vi "DI&AO.vi"() -> ()   [LabVIEW 2016]
uses:
  <vilib>/rvi/Emulation/niFpgaGetClockAttributes.vi
  <vilib>/rvi/Emulation/niFpgaSctlEmulationGetInTimedLoop.vi
  <vilib>/rvi/Emulation/niFpgaEmulationReportErrorSimple.vi
  <vilib>/rvi/eio/common/nirviEmuTemplateMethod_errors.vi
  <vilib>/rvi/Emulation/niFpgaCriticalErrorInLSC.vi
  <vilib>/eio/EIONode/EIONode.xnode
panel:
  out "Boolean array":bool[](array[boolean])
  out "Mod2/DIO31:0":u32
  in  "Mod4/AO7":fxp<+/-,20,5>
  in  "Mod4/AO6":fxp<+/-,20,5>
  in  "Mod4/AO5":fxp<+/-,20,5>
  in  "Mod4/AO4":fxp<+/-,20,5>
  in  "Mod4/AO3":fxp<+/-,20,5>
  in  "Mod4/AO2":fxp<+/-,20,5>
  in  "Mod4/AO1":fxp<+/-,20,5>
  in  "Mod4/AO0":fxp<+/-,20,5>
  in  "Mod4/AO15":fxp<+/-,20,5>
  in  "Mod4/AO14":fxp<+/-,20,5>
  in  "Mod4/AO13":fxp<+/-,20,5>
  in  "Mod4/AO12":fxp<+/-,20,5>
  in  "Mod4/AO11":fxp<+/-,20,5>
  in  "Mod4/AO10":fxp<+/-,20,5>
  in  "Mod4/AO9":fxp<+/-,20,5>
  in  "Mod4/AO8":fxp<+/-,20,5>
  out "Mod2/DIO31":bool
  out "Mod2/DIO30":bool
  out "Mod2/DIO29":bool
  out "Mod2/DIO28":bool
  out "Mod2/DIO27":bool
  out "Mod2/DIO26":bool
  out "Mod2/DIO25":bool
  out "Mod2/DIO24":bool
  out "Mod2/DIO23":bool
  out "Mod2/DIO22":bool
  out "Mod2/DIO21":bool
  out "Mod2/DIO20":bool
  out "Mod2/DIO19":bool
  out "Mod2/DIO18":bool
  out "Mod2/DIO17":bool
  out "Mod2/DIO16":bool
  out "Mod2/DIO15":bool
  out "Mod2/DIO14":bool
  out "Mod2/DIO13":bool
  out "Mod2/DIO12":bool
  out "Mod2/DIO11":bool
  out "Mod2/DIO10":bool
  out "Mod2/DIO9":bool
  out "Mod2/DIO8":bool
  out "Mod2/DIO7":bool
  out "Mod2/DIO6":bool
  out "Mod2/DIO5":bool
  out "Mod2/DIO4":bool
  out "Mod2/DIO3":bool
  out "Mod2/DIO2":bool
  out "Mod2/DIO1":bool
  out "Mod2/DIO0":bool
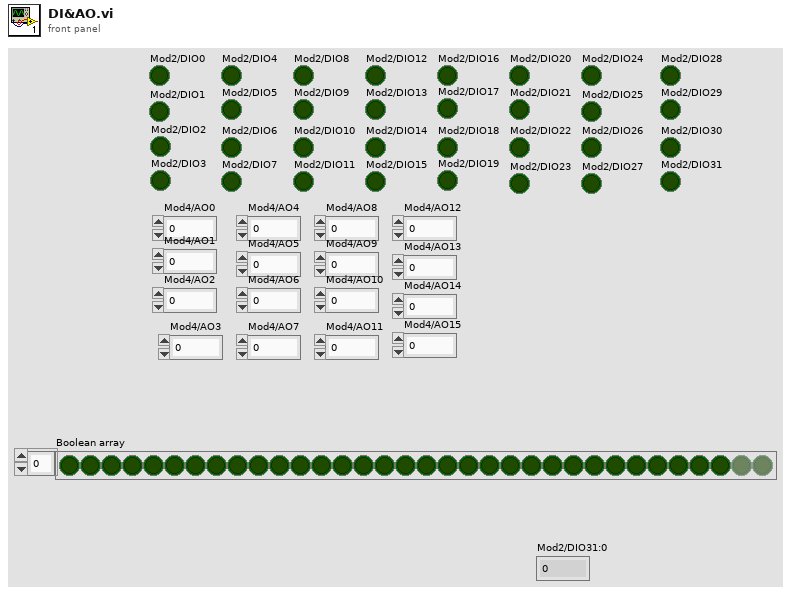
[diagram p1: front panel]
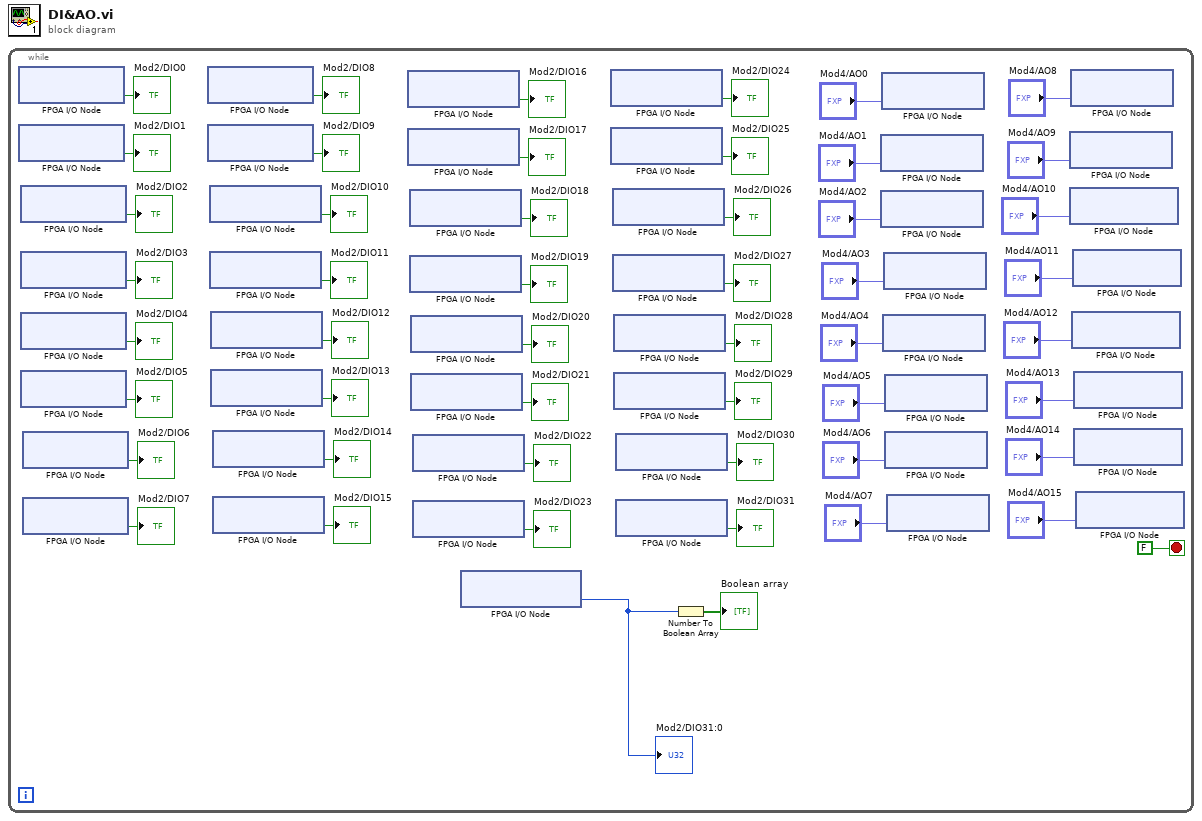
[diagram p0: block diagram]
diagram:
  n1 = while {
    stop <- FALSE stop-if-true
    n2 = xnode "FPGA I/O Node"() -> ("Mod2/DIO0"=→"Mod2/DIO0":bool)  [unwired: 1 in, 1 out]
    n3 = xnode "FPGA I/O Node"() -> ("Mod2/DIO1"=→"Mod2/DIO1":bool)  [unwired: 1 in, 1 out]
    n4 = xnode "FPGA I/O Node"() -> ("Mod2/DIO2"=→"Mod2/DIO2":bool)  [unwired: 1 in, 1 out]
    n5 = xnode "FPGA I/O Node"() -> ("Mod2/DIO3"=→"Mod2/DIO3":bool)  [unwired: 1 in, 1 out]
    n6 = xnode "FPGA I/O Node"() -> ("Mod2/DIO4"=→"Mod2/DIO4":bool)  [unwired: 1 in, 1 out]
    n7 = xnode "FPGA I/O Node"() -> ("Mod2/DIO5"=→"Mod2/DIO5":bool)  [unwired: 1 in, 1 out]
    n8 = xnode "FPGA I/O Node"() -> ("Mod2/DIO6"=→"Mod2/DIO6":bool)  [unwired: 1 in, 1 out]
    n9 = xnode "FPGA I/O Node"() -> ("Mod2/DIO7"=→"Mod2/DIO7":bool)  [unwired: 1 in, 1 out]
    n10 = xnode "FPGA I/O Node"() -> ("Mod2/DIO8"=→"Mod2/DIO8":bool)  [unwired: 1 in, 1 out]
    n11 = xnode "FPGA I/O Node"() -> ("Mod2/DIO9"=→"Mod2/DIO9":bool)  [unwired: 1 in, 1 out]
    n12 = xnode "FPGA I/O Node"() -> ("Mod2/DIO10"=→"Mod2/DIO10":bool)  [unwired: 1 in, 1 out]
    n13 = xnode "FPGA I/O Node"() -> ("Mod2/DIO11"=→"Mod2/DIO11":bool)  [unwired: 1 in, 1 out]
    n14 = xnode "FPGA I/O Node"() -> ("Mod2/DIO12"=→"Mod2/DIO12":bool)  [unwired: 1 in, 1 out]
    n15 = xnode "FPGA I/O Node"() -> ("Mod2/DIO13"=→"Mod2/DIO13":bool)  [unwired: 1 in, 1 out]
    n16 = xnode "FPGA I/O Node"() -> ("Mod2/DIO14"=→"Mod2/DIO14":bool)  [unwired: 1 in, 1 out]
    n17 = xnode "FPGA I/O Node"() -> ("Mod2/DIO15"=→"Mod2/DIO15":bool)  [unwired: 1 in, 1 out]
    n18 = xnode "FPGA I/O Node"() -> ("Mod2/DIO16"=→"Mod2/DIO16":bool)  [unwired: 1 in, 1 out]
    n19 = xnode "FPGA I/O Node"() -> ("Mod2/DIO17"=→"Mod2/DIO17":bool)  [unwired: 1 in, 1 out]
    n20 = xnode "FPGA I/O Node"() -> ("Mod2/DIO18"=→"Mod2/DIO18":bool)  [unwired: 1 in, 1 out]
    n21 = xnode "FPGA I/O Node"() -> ("Mod2/DIO19"=→"Mod2/DIO19":bool)  [unwired: 1 in, 1 out]
    n22 = xnode "FPGA I/O Node"() -> ("Mod2/DIO20"=→"Mod2/DIO20":bool)  [unwired: 1 in, 1 out]
    n23 = xnode "FPGA I/O Node"() -> ("Mod2/DIO21"=→"Mod2/DIO21":bool)  [unwired: 1 in, 1 out]
    n24 = xnode "FPGA I/O Node"() -> ("Mod2/DIO22"=→"Mod2/DIO22":bool)  [unwired: 1 in, 1 out]
    n25 = xnode "FPGA I/O Node"() -> ("Mod2/DIO23"=→"Mod2/DIO23":bool)  [unwired: 1 in, 1 out]
    n26 = xnode "FPGA I/O Node"() -> ("Mod2/DIO31:0"=w2:u32)  [unwired: 1 in, 1 out]
    "Mod2/DIO31:0" <- w2
    n27 = xnode "FPGA I/O Node"() -> ("Mod2/DIO24"=→"Mod2/DIO24":bool)  [unwired: 1 in, 1 out]
    n28 = xnode "FPGA I/O Node"() -> ("Mod2/DIO25"=→"Mod2/DIO25":bool)  [unwired: 1 in, 1 out]
    n29 = xnode "FPGA I/O Node"() -> ("Mod2/DIO26"=→"Mod2/DIO26":bool)  [unwired: 1 in, 1 out]
    n30 = xnode "FPGA I/O Node"() -> ("Mod2/DIO27"=→"Mod2/DIO27":bool)  [unwired: 1 in, 1 out]
    n31 = xnode "FPGA I/O Node"() -> ("Mod2/DIO28"=→"Mod2/DIO28":bool)  [unwired: 1 in, 1 out]
    n32 = xnode "FPGA I/O Node"() -> ("Mod2/DIO29"=→"Mod2/DIO29":bool)  [unwired: 1 in, 1 out]
    n33 = xnode "FPGA I/O Node"() -> ("Mod2/DIO30"=→"Mod2/DIO30":bool)  [unwired: 1 in, 1 out]
    n34 = xnode "FPGA I/O Node"() -> ("Mod2/DIO31"=→"Mod2/DIO31":bool)  [unwired: 1 in, 1 out]
    n35 = Number To Boolean Array(number=w2) -> (Boolean array=→"Boolean array":bool[])
    n36 = xnode "FPGA I/O Node"("Mod4/AO1"="Mod4/AO1") -> ()  [unwired: 1 in, 1 out]
    n37 = xnode "FPGA I/O Node"("Mod4/AO2"="Mod4/AO2") -> ()  [unwired: 1 in, 1 out]
    n38 = xnode "FPGA I/O Node"("Mod4/AO0"="Mod4/AO0") -> ()  [unwired: 1 in, 1 out]
    n39 = xnode "FPGA I/O Node"("Mod4/AO4"="Mod4/AO4") -> ()  [unwired: 1 in, 1 out]
    n40 = xnode "FPGA I/O Node"("Mod4/AO3"="Mod4/AO3") -> ()  [unwired: 1 in, 1 out]
    n41 = xnode "FPGA I/O Node"("Mod4/AO5"="Mod4/AO5") -> ()  [unwired: 1 in, 1 out]
    n42 = xnode "FPGA I/O Node"("Mod4/AO6"="Mod4/AO6") -> ()  [unwired: 1 in, 1 out]
    n43 = xnode "FPGA I/O Node"("Mod4/AO7"="Mod4/AO7") -> ()  [unwired: 1 in, 1 out]
    n44 = xnode "FPGA I/O Node"("Mod4/AO9"="Mod4/AO9") -> ()  [unwired: 1 in, 1 out]
    n45 = xnode "FPGA I/O Node"("Mod4/AO10"="Mod4/AO10") -> ()  [unwired: 1 in, 1 out]
    n46 = xnode "FPGA I/O Node"("Mod4/AO8"="Mod4/AO8") -> ()  [unwired: 1 in, 1 out]
    n47 = xnode "FPGA I/O Node"("Mod4/AO12"="Mod4/AO12") -> ()  [unwired: 1 in, 1 out]
    n48 = xnode "FPGA I/O Node"("Mod4/AO11"="Mod4/AO11") -> ()  [unwired: 1 in, 1 out]
    n49 = xnode "FPGA I/O Node"("Mod4/AO13"="Mod4/AO13") -> ()  [unwired: 1 in, 1 out]
    n50 = xnode "FPGA I/O Node"("Mod4/AO14"="Mod4/AO14") -> ()  [unwired: 1 in, 1 out]
    n51 = xnode "FPGA I/O Node"("Mod4/AO15"="Mod4/AO15") -> ()  [unwired: 1 in, 1 out]
  }
